vi "exampleloop_dirty.vi"() -> ()   [LabVIEW 2011]
uses:
  Kelvinox drivers/ITCAPPS - Copie.LLB/ITCSignal.ctl
  Kelvinox drivers/ITCAPPS - Copie.LLB/ITCSignals.ctl
  stopButton.vi
panel:
  in  "Refresh Rate [ms]":i32=1000 min=0
  out "Current sweep":dbl
  out "ITC ref":T1={"ITC"=0, "Signal"=enum."Sensor 3"}
  in  "Cancel run":bool
  out "DAC number":u8
  out "DAC":refnum<visa-resource-name>
  out "K2400 2":refnum<visa-resource-name>
  out "Lockin1":refnum<visa-resource-name>
  out "K2400 1":refnum<visa-resource-name>
  out "Priority type array":string[](array[string])
  out "Total sweep sequence":dbl[][](array[numeric])
  in  "Device Cluster":T3={"K2400 1"="", "K2400_1"=FALSE, "K2400 2"="", "K2400_2"=FALSE, "Lockin1"="", "Lockin1 present"=FALSE, "Lockin2"="", "Lockin2 present"=FALSE, "TIC"="", "Tcontrol"="OFF", "DMM1"="", "DMM1"=FALSE, "DMM2"="", "DMM2"=FALSE, "DAC"="", "DAC present"=FALSE, "DAC number"=0, "Bfield query"=FALSE, "Wvlen query"=FALSE, "ITC signal"={"ITC"=0, "Signal"=enum."Sensor 1"}}
  in  "Tab Control":T4(tab)
  in  "Loop Cluster":T5
  in  "START":bool
  in  "genTotalSequence":bool
  in  "Conversion Factor Fix\n1 V = ??":dbl=1.0
  in  "Fix type":string(combo)
  in  "Sweep Bias":dbl[](array[numeric])
  in  "Fix Bias":dbl[](array[numeric])
  in  "Priority sweep":i32=2
  in  "Priority fix":i32=2
  in  "sweep start [V]":dbl=-1.0 min=-200.0 max=200.0
  in  "sweep stop [V]":dbl=-5.0 min=-250.0 max=250.0
  in  "Nb steps":i32=800
  in  "sweep stop 2 [V]":dbl min=-250.0 max=250.0
  in  "Nb steps 2":i32
  in  "Nb Sweep":i32=1
  in  "Nb steps fix2":i32
  in  "Fix stop 2":dbl min=-250.0 max=250.0
  in  "Nb steps fix":i32=800
  in  "Fix stop":dbl=-5.0 min=-250.0 max=250.0
  in  "Fix start":dbl=-1.0 min=-200.0 max=200.0
  in  "genSweepArray":bool
  in  "genFixArray":bool
  in  "Sweep Instrument":string(combo)
  in  "Conversion Factor Sweep\n1 V = ??":dbl=1.0
  in  "Fix Instrument":string(combo)
  in  "Sweep type":string(combo)
  in  "T [K]":dbl[](array[numeric])
  in  "Priority T":i32=2
  in  "T stop [K] 2":dbl=-1.0 min=-200.0 max=200.0
  in  "Nb T steps 2":i32=800
  in  "Nb T steps":i32=800
  in  "T stop [K]":dbl=-1.0 min=-200.0 max=200.0
  in  "T start [K]":dbl=-1.0 min=-200.0 max=200.0
  in  "genTarray":bool
  in  "B [T]":dbl[](array[numeric])
  in  "Priority B":i32=2
  in  "B start [T]":dbl=-1.0 min=-200.0 max=200.0
  in  "B stop [T]":dbl=-1.0 min=-200.0 max=200.0
  in  "Rate [T/min]":dbl=-1.0 min=-200.0 max=200.0
  in  "Nb B steps":i32=800
  in  "Nb B steps 2":i32=800
  in  "B stop [T] 2":dbl=-1.0 min=-200.0 max=200.0
  in  "GenBarray":bool
  in  "File Basename":string
  out "Bias factor":dbl
  in  "SD bias [V]":dbl=-1.0 min=-200.0 max=200.0
  in  "Gain Cluster":T6={"Vsd"="Gate", "I 2probe 2"="Gate", "Vxy"="Gate", "Vxx"="Gate", "I leak BG"="Gate", "I leak TG"="Gate", "I Gain 1"=1000000.0, "V Gain 1"=1.0, "conversion factor BG"=1.0, "Vin / Vout 1"=1.0, "V Gain 2"=1.0, "Vin / Vout 2"=1.0, "V Gain 3"=1.0, "Vin / Vout 3"=1.0, "I Gain 2"=1000000.0, "I Gain 3"=1000000.0, "V BG"="Gate", "V TG"="Gate", "conversion factor TG"=1.0, "Vin / Vout 4"=1.0, "Vin / Vout 5"=1.0, "Manual Gain 1"=1.0, "Manual Gain 2"=1.0, "Manual Gain 3"=1.0} {"conversion factor TG" items=["1 V/V"=1.0, "4 V/V"=4.0, "15 V/V"=15.0, "30 V/V"=30.0, "45 V/V"=45.0]; "I Gain 3" items=["1"=1.0, "10"=10.0, "100"=100.0, "1K"=1000.0, "10K"=10000.0, "100K"=100000.0, "1M"=1000000.0, "10M"=10000000.0, "100M"=100000000.0, "1G"=1000000000.0]; "I Gain 2" items=["1"=1.0, "10"=10.0, "100"=100.0, "1K"=1000.0, "10K"=10000.0, "100K"=100000.0, "1M"=1000000.0, "10M"=10000000.0, "100M"=100000000.0, "1G"=1000000000.0]; "V Gain 3" items=["1"=1.0, "10"=10.0, "100"=100.0, "1K"=1000.0, "10K"=10000.0]; "V Gain 2" items=["1"=1.0, "10"=10.0, "100"=100.0, "1K"=1000.0, "10K"=10000.0]; "conversion factor BG" items=["1 V/V"=1.0, "4 V/V"=4.0, "15 V/V"=15.0, "30 V/V"=30.0, "45 V/V"=45.0]; "V Gain 1" items=["1"=1.0, "10"=10.0, "100"=100.0, "1K"=1000.0, "10K"=10000.0]; "I Gain 1" items=["1"=1.0, "10"=10.0, "100"=100.0, "1K"=1000.0, "10K"=10000.0, "100K"=100000.0, "1M"=1000000.0, "10M"=10000000.0, "100M"=100000000.0, "1G"=1000000000.0]}
  in  "Nb steps Increase 2":dbl=10.0
  in  "Gate Increase 2 (V)":dbl=0.1
  in  "Nb steps Increase":dbl=10.0
  in  "Gate Increase (V)":dbl=-0.1
  in  "Sweep back to zero":bool
  out "x .or. y?":bool
  in  "Step Delay (ms)":dbl=1000.0
  out "Total Progress":dbl(slide) scale=0.0..1.0
  in  "Nb Loop":i32
  out "Nb Loop Indicator":i32=2
  out "Nb Sweep Indicator":i32=3
  out "conversion factor sweep":dbl(ring)=1.0 items=["1 V/V"=1.0, "4 V/V"=4.0, "15 V/V"=15.0, "30 V/V"=30.0, "45 V/V"=45.0]
  in  "stop":bool
  in  "V step [V]":dbl=0.001
  in  "Folder Name":path=path "D:/users/marc/20180122_LiIon_EL/Freezing02/OutputHighT002p2.dat"
  # "Magnetic Field"
  # "Wavelength"
  # "IV Sweep Setting"
  # "IV Fix Setting"
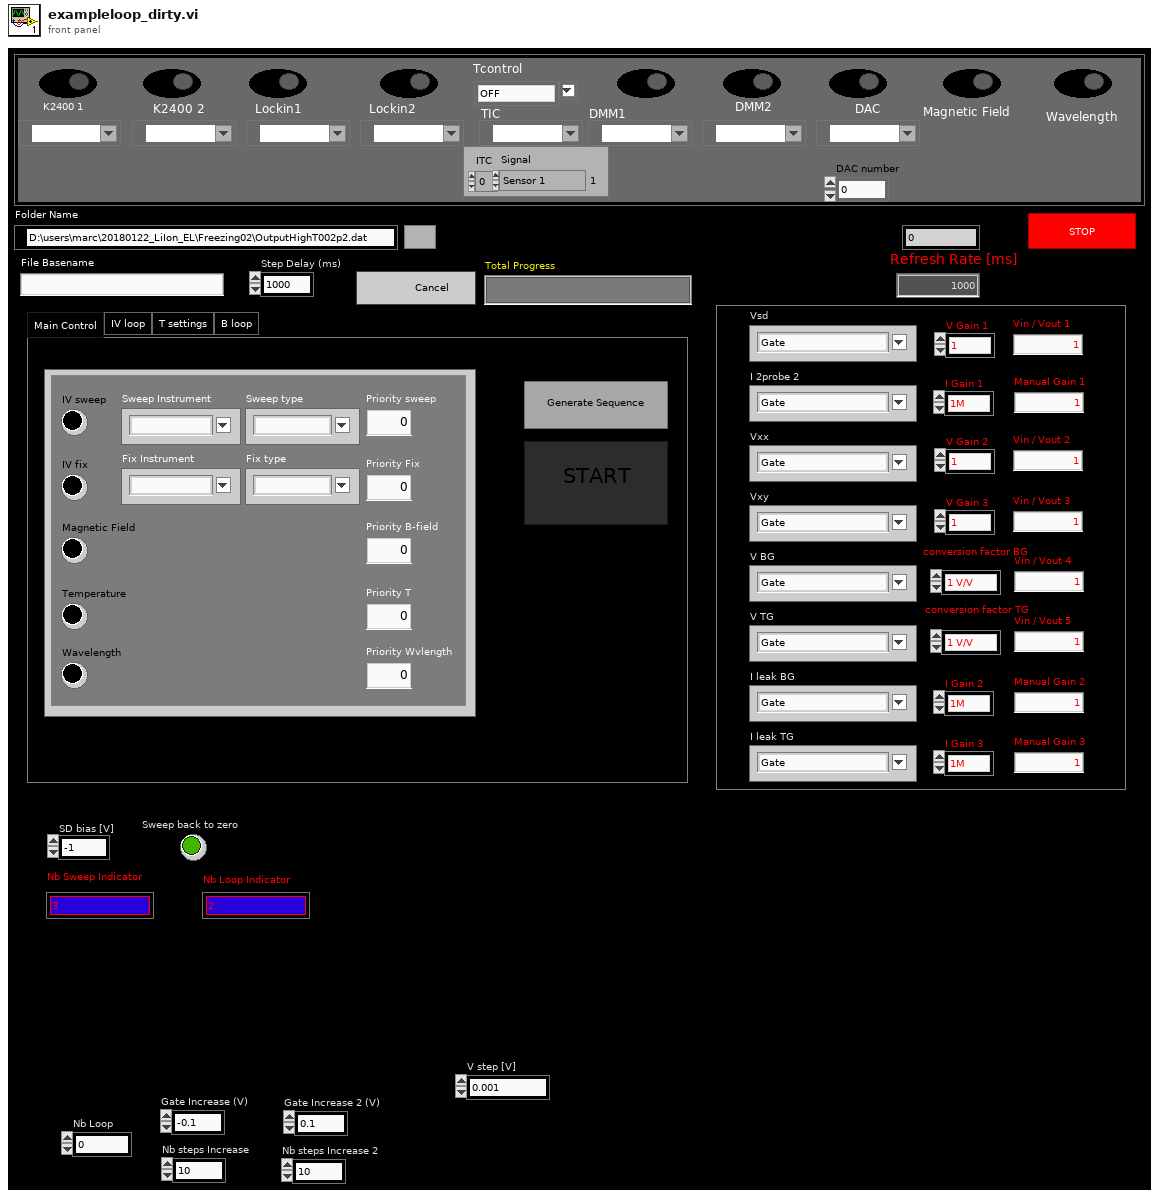
[diagram p1: front panel]
types:
  T1 = typedef "ITCSignal.ctl" = cluster{"ITC":u16, "Signal":T2}
  T2 = typedef "ITCSignals.ctl" = enum16{"Setpoint", "Sensor 1", "Sensor 2", "Sensor 3", "Needle Valve %", "Heater %"}
  T3 = cluster{"K2400 1":refnum<visa-resource-name>, "K2400_1":bool, "K2400 2":refnum<visa-resource-name>, "K2400_2":bool, "Lockin1":refnum<visa-resource-name>, "Lockin1 present":bool, "Lockin2":refnum<visa-resource-name>, "Lockin2 present":bool, "TIC":refnum<visa-resource-name>, "Tcontrol":string, "DMM1":refnum<visa-resource-name>, "DMM1":bool, "DMM2":refnum<visa-resource-name>, "DMM2":bool, "DAC":refnum<visa-resource-name>, "DAC present":bool, "DAC number":u8, "Bfield query":bool, "Wvlen query":bool, "ITC signal":T1}
  T4 = enum32{"Main Control", "IV loop", "T settings", "B loop"}
  T5 = cluster{"Sweep Instrument":string, "Sweep type":string, "Fix Instrument":string, "Fix type":string, "IV sweep":bool, "IV fix":bool, "Magnetic Field":bool, "Temperature":bool, "Wavelength":bool, "Priority sweep":dbl, "Priority Fix":dbl, "Priority B-field":dbl, "Priority T":dbl, "Priority Wvlength":dbl}
  T6 = cluster{"Vsd":string, "I 2probe 2":string, "Vxy":string, "Vxx":string, "I leak BG":string, "I leak TG":string, "I Gain 1":dbl, "V Gain 1":dbl, "conversion factor BG":dbl, "Vin / Vout 1":dbl, "V Gain 2":dbl, "Vin / Vout 2":dbl, "V Gain 3":dbl, "Vin / Vout 3":dbl, "I Gain 2":dbl, "I Gain 3":dbl, "V BG":string, "V TG":string, "conversion factor TG":dbl, "Vin / Vout 4":dbl, "Vin / Vout 5":dbl, "Manual Gain 1":dbl, "Manual Gain 2":dbl, "Manual Gain 3":dbl}
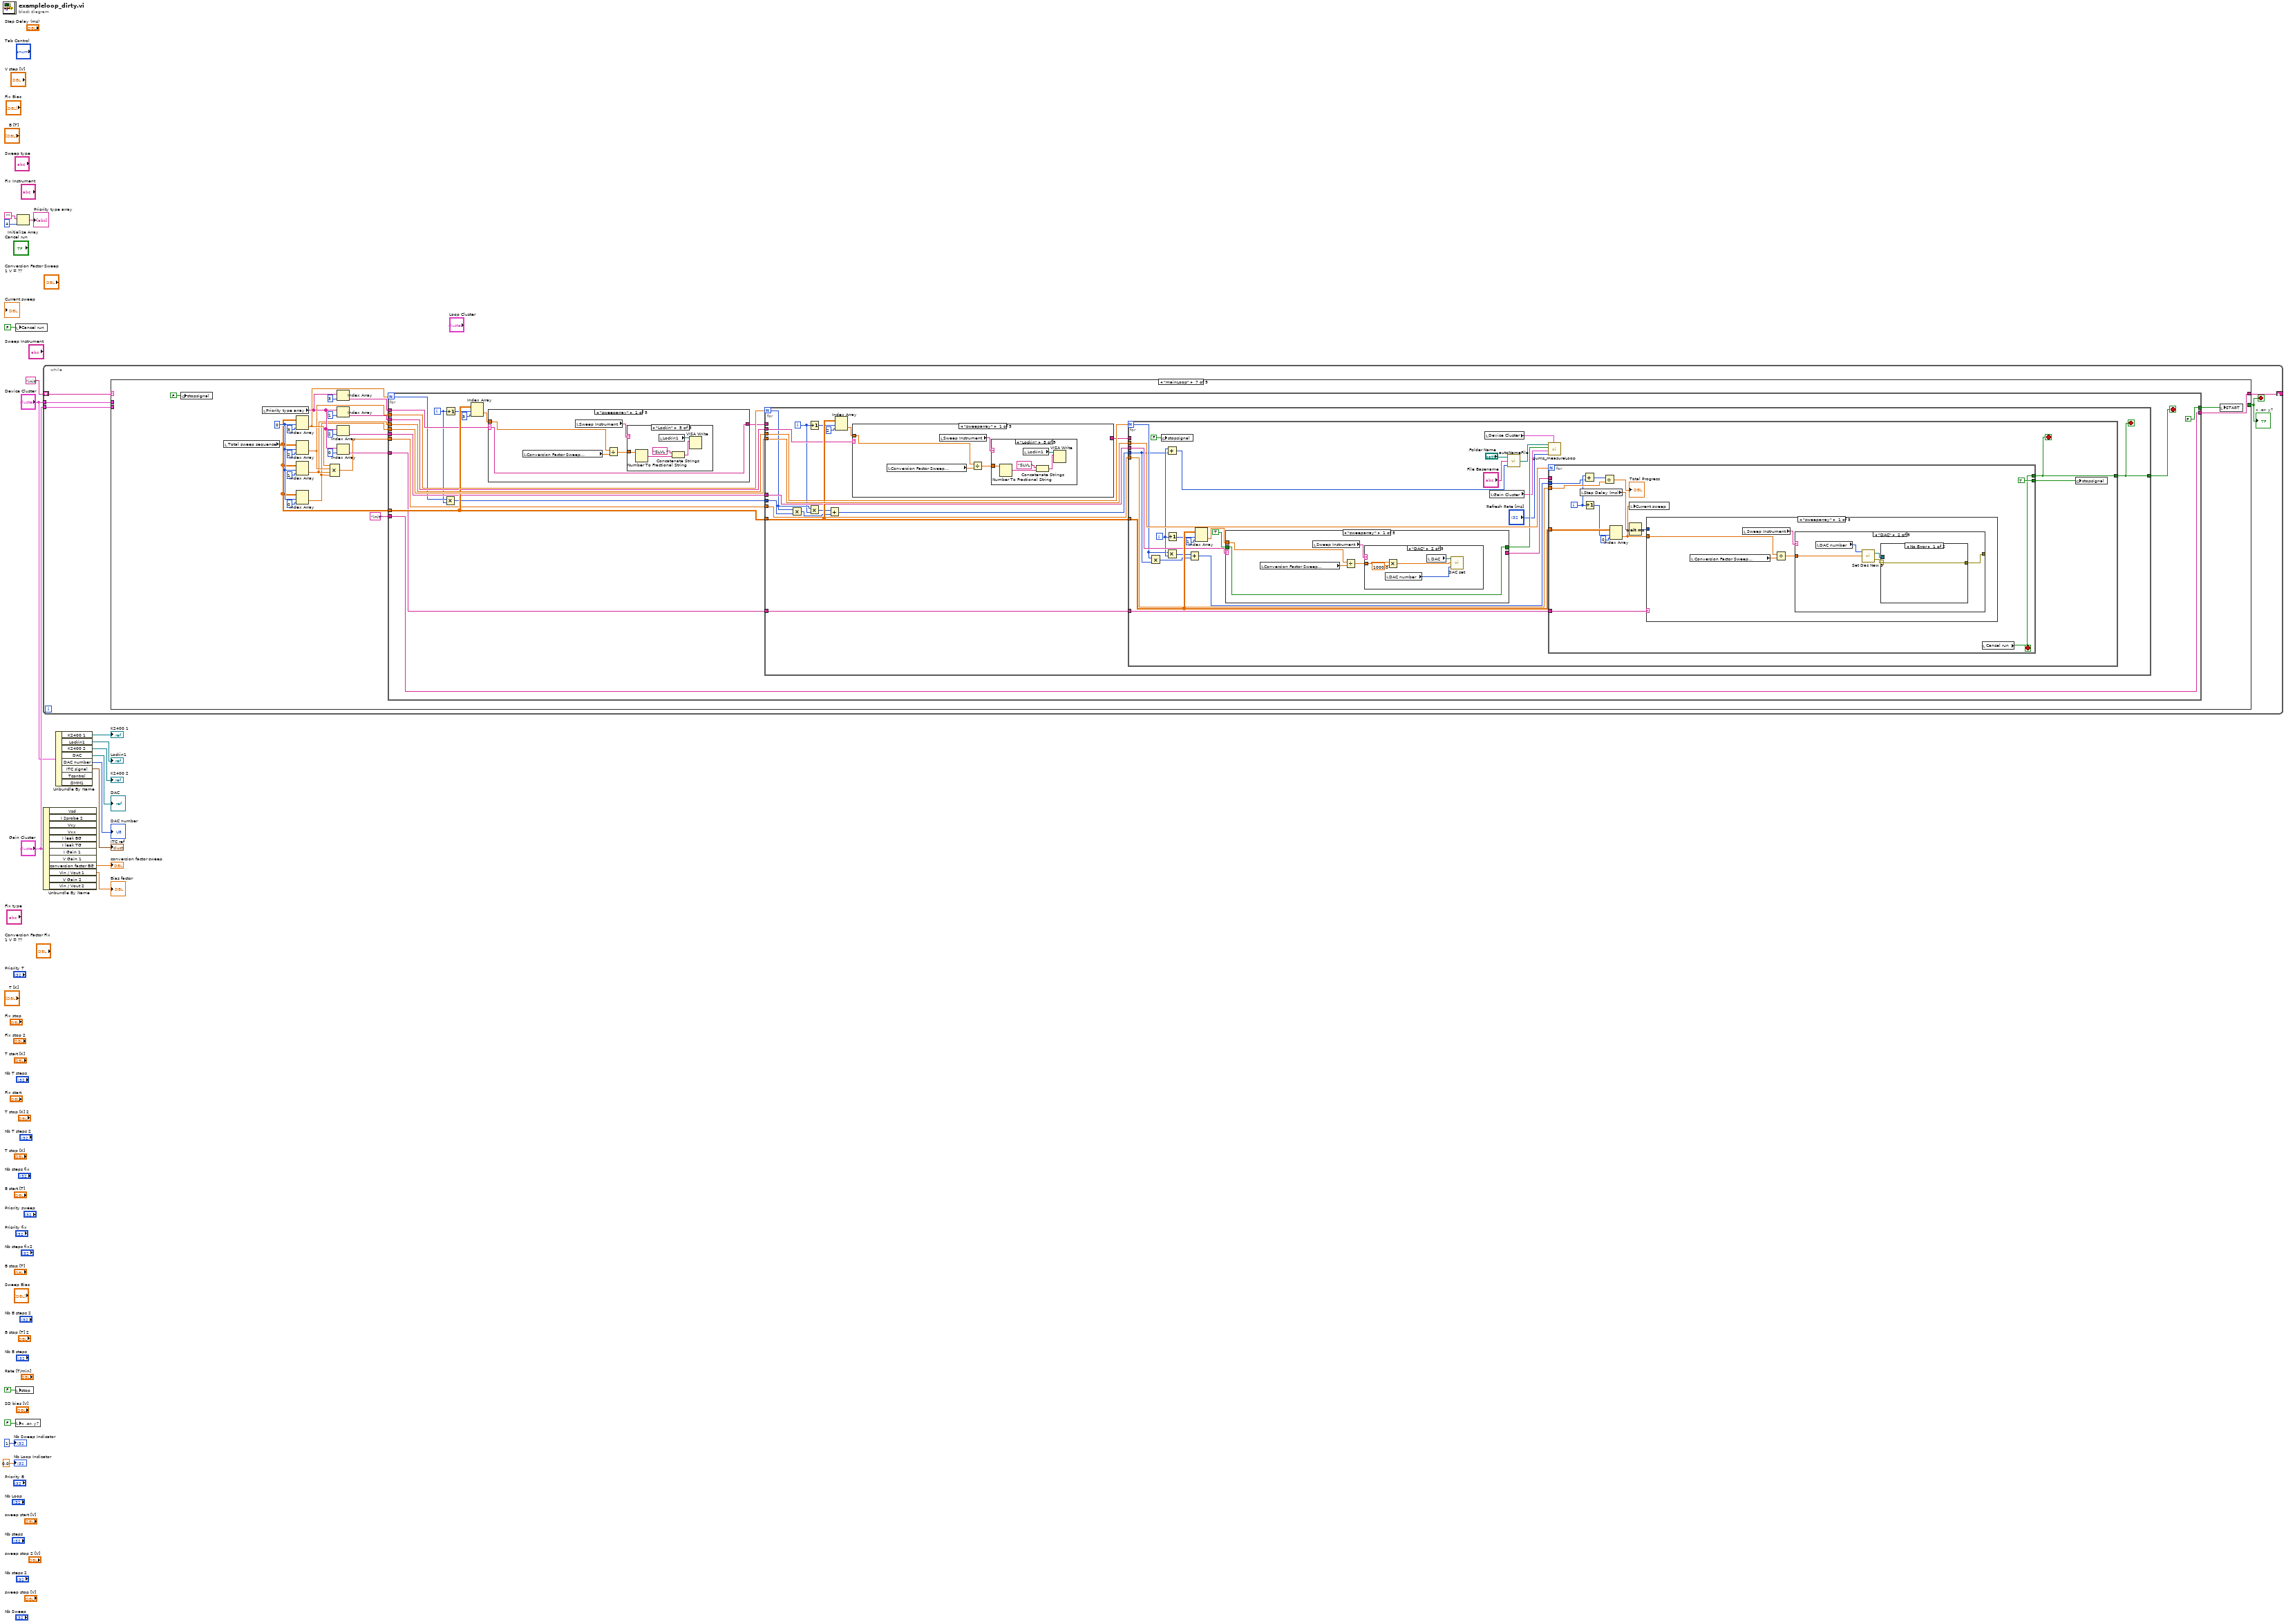
[diagram p0: block diagram]
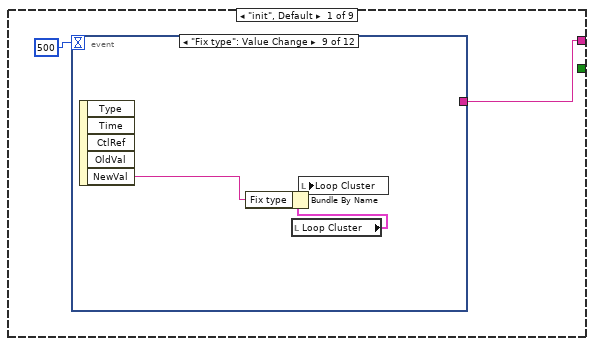
[diagram p2: hidden frame]
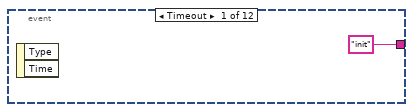
[diagram p3: hidden frame]
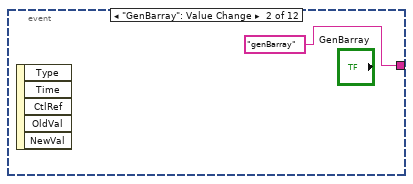
[diagram p4: hidden frame]
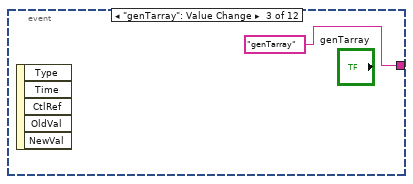
[diagram p5: hidden frame]
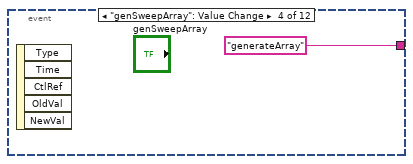
[diagram p6: hidden frame]
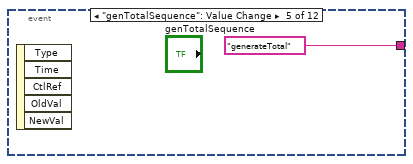
[diagram p7: hidden frame]
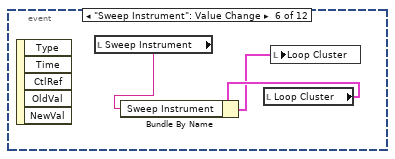
[diagram p8: hidden frame]
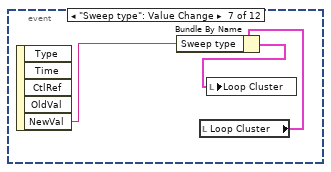
[diagram p9: hidden frame]
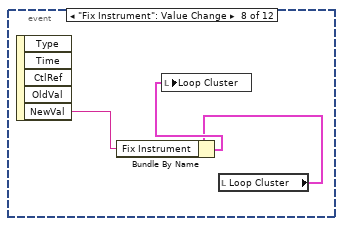
[diagram p10: hidden frame]
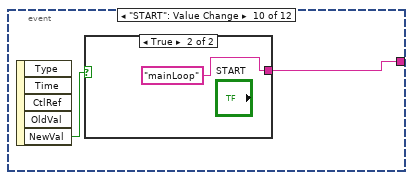
[diagram p11: hidden frame]
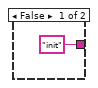
[diagram p12: hidden frame]
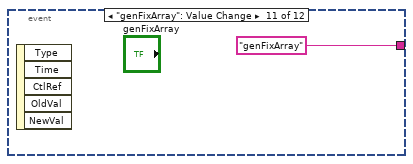
[diagram p13: hidden frame]
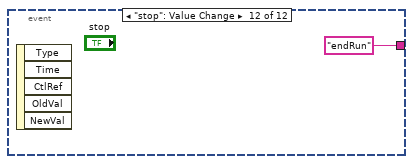
[diagram p14: hidden frame]
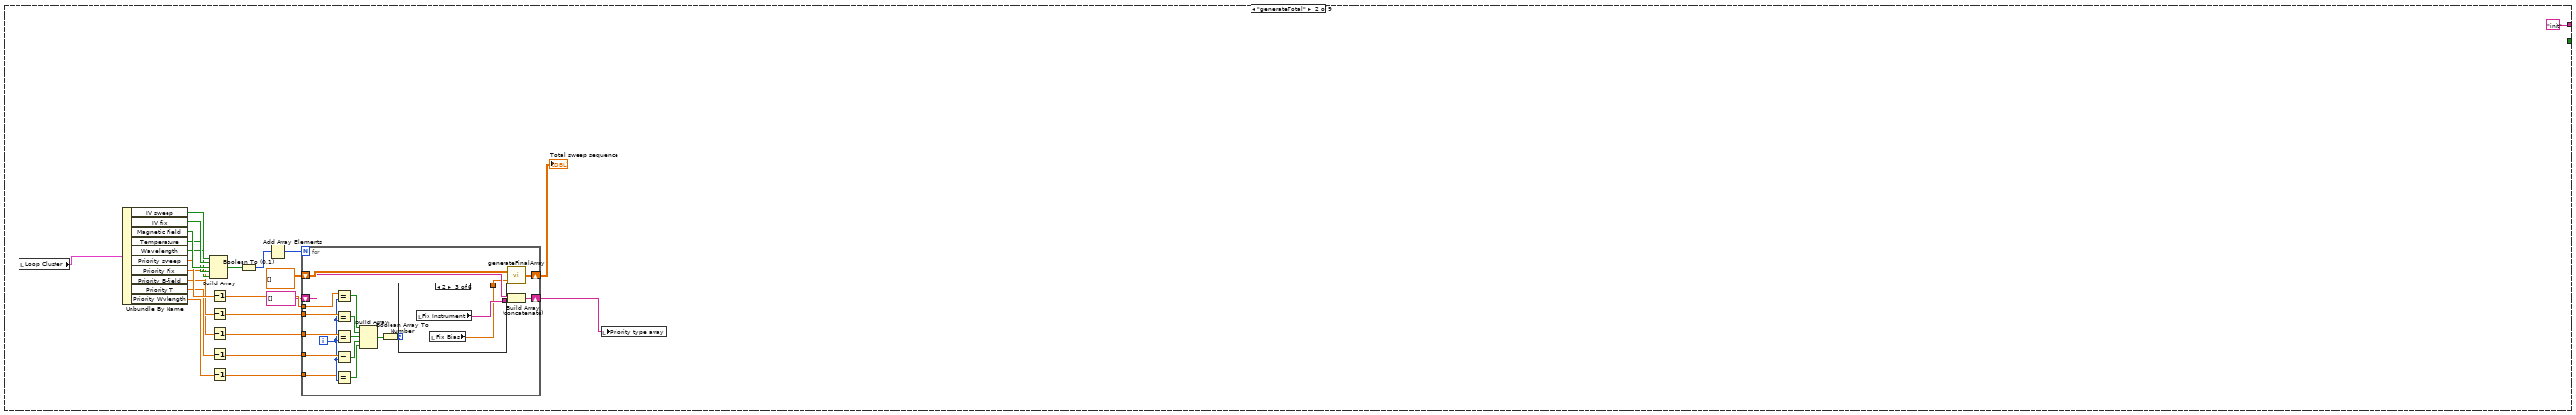
[diagram p15: hidden frame]
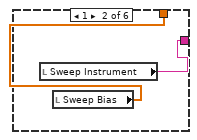
[diagram p17: hidden frame]
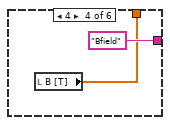
[diagram p18: hidden frame]
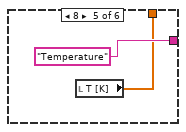
[diagram p19: hidden frame]
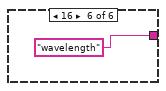
[diagram p20: hidden frame]
diagram:
  n1 = local write "Cancel run"(FALSE ("Cancel run")) -> ()
  n2 = local write "stop"(FALSE ("stop")) -> ()
  n3 = local write "x .or. y?"(FALSE ("x .or. y?")) -> ()
  n4 = Initialize Array("", 4 ("dimension size")) -> (→"Priority type array":string[])
  n5 = while {
    shift-right: [w20] -> _
    shift-left: "init" -> [w24]
    tunnel: "Gain Cluster" -> [w22]
    tunnel: "Device Cluster" -> [w21]
    stop <- w23 stop-if-true
    n6 = case shown="\"mainLoop\"" w24 {
      tunnel: [_ _ _ _ _ _ _ _ TRUE] -> w23
      tunnel: [w25 "init" "init" "init" "init" "init" w189 "generateArray" ""] -> w20
      tunnel: w22 -> [_ _ _ _ _ _ _ _ _]
      tunnel: w21 -> [_ _ _ _ _ _ _ _ _]
      frame "init", Default {
        n7 = event shown="[8] \"Fix type\": Value Change" {
          selector: _ -> [_ _ _ _ _ _ _ _ _ _ _ _]
          dyn-events: _ -> [_ _ _ _ _ _ _ _ _ _ _ _]
          timeout: 500 -> [_ _ _ _ _ _ _ _ _ _ _ _]
          tunnel: ["init" "genBarray" "genTarray" "generateArray" "generateTotal" _ _ _ _ w44 "genFixArray" "endRun"] -> w25
          event Timeout {
            n8 = event-data() -> ()  [unwired: 1 in, 2 out]
          }
          event "GenBarray": Value Change {
            n9 = event-data() -> ()  [unwired: 1 in, 5 out]
          }
          event "genTarray": Value Change {
            n10 = event-data() -> ()  [unwired: 1 in, 5 out]
          }
          event "genSweepArray": Value Change {
            n11 = event-data() -> ()  [unwired: 1 in, 5 out]
          }
          event "genTotalSequence": Value Change {
            n12 = event-data() -> ()  [unwired: 1 in, 5 out]
          }
          event "Sweep Instrument": Value Change {
            n13 = event-data() -> ()  [unwired: 1 in, 5 out]
            n14 = local read "Sweep Instrument"() -> (w33:string)
            n15 = local read "Loop Cluster"() -> (w34:T5)
            n16 = Bundle By Name(cluster=w34, "Sweep Instrument"=w33) -> (w32:T5)
            n17 = local write "Loop Cluster"(w32) -> ()
          }
          event "Sweep type": Value Change {
            n18 = event-data() -> ("NewVal"=w35:string)  [unwired: 1 in, 4 out]
            n19 = local read "Loop Cluster"() -> (w37:T5)
            n20 = Bundle By Name(cluster=w37, "Sweep type"=w35) -> (w36:T5)
            n21 = local write "Loop Cluster"(w36) -> ()
          }
          event "Fix Instrument": Value Change {
            n22 = event-data() -> ("NewVal"=w38:string)  [unwired: 1 in, 4 out]
            n23 = local read "Loop Cluster"() -> (w39:T5)
            n24 = Bundle By Name(cluster=w39, "Fix Instrument"=w38) -> (w40:T5)
            n25 = local write "Loop Cluster"(w40) -> ()
          }
          event "Fix type": Value Change {
            n26 = event-data() -> ("NewVal"=w43:string)  [unwired: 1 in, 4 out]
            n27 = local read "Loop Cluster"() -> (w42:T5)
            n28 = Bundle By Name(cluster=w42, "Fix type"=w43) -> (w41:T5)
            n29 = local write "Loop Cluster"(w41) -> ()
          }
          event "START": Value Change {
            n30 = event-data() -> ("NewVal"=w45:bool)  [unwired: 1 in, 4 out]
            n31 = case shown="True" w45 {
              tunnel: ["init" "mainLoop"] -> w44
              frame False {
              }
              frame True {
              }
            }
          }
          event "genFixArray": Value Change {
            n32 = event-data() -> ()  [unwired: 1 in, 5 out]
          }
          event "stop": Value Change {
            n33 = event-data() -> ()  [unwired: 1 in, 5 out]
          }
        }
      }
      frame "generateTotal" {
        n34 = local read "Loop Cluster"() -> (w52:T5)
        n35 = Unbundle By Name(w52) -> ("IV sweep"=w72:bool, "IV fix"=w71:bool, "Magnetic Field"=w70:bool, "Temperature"=w69:bool, "Wavelength"=w68:bool, "Priority sweep"=w63:dbl, "Priority Fix"=w62:dbl, "Priority B-field"=w61:dbl, "Priority T"=w60:dbl, "Priority Wvlength"=w55:dbl)
        n36 = Build Array(w72, w71, w70, w69, w68) -> (w66:bool[])
        n37 = Decrement(x=w63) -> (x-1=w56:dbl)
        n38 = Decrement(x=w62) -> (x-1=w57:dbl)
        n39 = Decrement(x=w61) -> (x-1=w58:dbl)
        n40 = Decrement(x=w60) -> (x-1=w59:dbl)
        n41 = Decrement(x=w55) -> (x-1=w54:dbl)
        n42 = Boolean To (0,1)(Boolean=w66) -> (0, 1=w67:i16[])
        n43 = Add Array Elements(numeric array=w67) -> (sum=w65:i16)
        n44 = for {
          N: w65 -> [_]
          shift-right: [w91] -> w51
          shift-left: dbl[][] [] ("Array In") -> [w92]
          tunnel: w59 -> [w88]
          tunnel: w58 -> [w89]
          tunnel: w57 -> [w90]
          tunnel: w56 -> [w82]
          tunnel: w54 -> [w84]
          shift-right: [w77] -> w50
          shift-left: string[] [] -> [w75]
          i -> [w85]
          n45 = Equal?(x=w82, y=w85) -> (x = y?=w81:bool)
          n46 = Equal?(x=w90, y=w85) -> (x = y?=w80:bool)
          n47 = Equal?(x=w89, y=w85) -> (x = y?=w79:bool)
          n48 = Equal?(x=w88, y=w85) -> (x = y?=w78:bool)
          n49 = Equal?(x=w84, y=w85) -> (x = y?=w83:bool)
          n50 = Build Array(w81, w80, w79, w78, w83) -> (w87:bool[])
          n51 = Boolean Array To Number(Boolean array=w87) -> (number=w86:u32)
          n52 = case shown="2" w86 {
            tunnel: [_ w94 w96 "Bfield" ("Fix Instrument") "Temperature" "wavelength"] -> w76
            tunnel: [_ w93 w95 w97 w99 _] -> w74
            frame 0, Default {
            }
            frame 1 {
              n53 = local read "Sweep Instrument"() -> (w94:string)
              n54 = local read "Sweep Bias"() -> (w93:dbl[])
            }
            frame 2 {
              n55 = local read "Fix Instrument"() -> (w96:string)
              n56 = local read "Fix Bias"() -> (w95:dbl[])
            }
            frame 4 {
              n57 = local read "B [T]"() -> (w97:dbl[])
            }
            frame 8 {
              n58 = local read "T [K]"() -> (w99:dbl[])
            }
            frame 16 {
            }
          }
          n59 = call "generateFinalArray.vi"("new array"=w74, "Array In"=w92) -> ("Array out"=w91:dbl[][])
          n60 = Build Array (concatenate)(w75, w76) -> (w77:string[])
        }
        "Total sweep sequence" <- w51
        n61 = local write "Priority type array"(w50) -> ()
      }
      frame "generateArray" {
        n62 = local read "Sweep Bias"() -> (w108:dbl[])
        n63 = local read "Nb Sweep"() -> (w109:i32)
        n64 = local read "Priority sweep"() -> (w102:i32)
        n65 = for {
          N: w109 -> [_]
          shift-right: [w113] -> w107
          shift-left: w108 -> [w112]
          n66 = local read "sweep stop 2 [V]"() -> (w115:dbl)
          n67 = local read "sweep start [V]"() -> (w116:dbl)
          n68 = local read "sweep stop [V]"() -> (w114:dbl)
          n69 = local read "Nb steps 2"() -> (w117:i32)
          n70 = local read "Nb steps"() -> (w118:i32)
          n71 = call "createLoopArray.vi"("Bgstop"=w114, "Bgstop2"=w115, "nbpoint1"=w118, "nbpoint2"=w117, "Bgstart"=w116) -> ("Outarray"=w111:dbl[])
          n72 = Build Array (concatenate)(w112, w111) -> (w113:dbl[])
        }
        n73 = local read "Priority type array"() -> (w106:string[])
        n74 = Decrement(x=w102) -> (x-1=w103:i32)
        n75 = Replace Array Subset(array=w106, new element="sweeparray" ("new element/subarray"), index=w103) -> (w105:string[])
        n76 = local write "Priority type array"(w105) -> ()
        n77 = local write "Sweep Bias"(w107) -> ()
      }
      frame "genFixArray" {
        n78 = local read "Priority fix"() -> (w119:i32)
        n79 = local read "Nb Sweep"() -> (w126:i32)
        n80 = local read "Fix Bias"() -> (w125:dbl[])
        n81 = local read "Priority type array"() -> (w123:string[])
        n82 = for {
          N: w126 -> [_]
          shift-right: [w130] -> w124
          shift-left: w125 -> [w129]
          n83 = local read "Nb steps fix2"() -> (w134:i32)
          n84 = local read "Nb steps fix"() -> (w135:i32)
          n85 = local read "Fix stop 2"() -> (w132:dbl)
          n86 = local read "Fix start"() -> (w133:dbl)
          n87 = local read "Fix stop"() -> (w131:dbl)
          n88 = call "createLoopArray.vi"("Bgstop"=w131, "Bgstop2"=w132, "nbpoint1"=w135, "nbpoint2"=w134, "Bgstart"=w133) -> ("Outarray"=w128:dbl[])
          n89 = Build Array (concatenate)(w129, w128) -> (w130:dbl[])
        }
        n90 = Decrement(x=w119) -> (x-1=w120:i32)
        n91 = Replace Array Subset(array=w123, new element="Fixarray" ("new element/subarray"), index=w120) -> (w122:string[])
        n92 = local write "Priority type array"(w122) -> ()
        n93 = local write "Fix Bias"(w124) -> ()
      }
      frame "genBarray" {
        n94 = local read "Priority B"() -> (w137:i32)
        n95 = local read "Priority type array"() -> (w140:string[])
        n96 = local read "Nb B steps 2"() -> (w143:i32)
        n97 = local read "B stop [T] 2"() -> (w145:dbl)
        n98 = local read "Nb B steps"() -> (w144:i32)
        n99 = local read "B start [T]"() -> (w147:dbl)
        n100 = local read "B stop [T]"() -> (w146:dbl)
        n101 = Decrement(x=w137) -> (x-1=w136:i32)
        n102 = Equal?(x=w137, y=1) -> (x = y?=w141:bool)
        n103 = case shown="True" w141 {
          tunnel: [w155 w156] -> w148
          tunnel: w147 -> [w154 w158]
          tunnel: w146 -> [w153 w157]
          tunnel: w145 -> [w152 _]
          tunnel: w144 -> [w151 _]
          tunnel: w143 -> [w150 _]
          frame False {
            n104 = call "createLoopArray.vi"("Bgstop"=w153, "Bgstop2"=w152, "nbpoint1"=w151, "nbpoint2"=w150, "Bgstart"=w154) -> ("Outarray"=w155:dbl[])
          }
          frame True {
            n105 = Build Array(w158, w157) -> (w156:dbl[])
          }
        }
        n106 = Replace Array Subset(array=w140, new element="Bfield" ("new element/subarray"), index=w136) -> (w139:string[])
        n107 = local write "Priority type array"(w139) -> ()
        n108 = local write "B [T]"(w148) -> ()
      }
      frame "genTarray" {
        n109 = local read "Priority T"() -> (w161:i32)
        n110 = local read "Priority type array"() -> (w163:string[])
        n111 = local read "Nb B steps 2"() -> (w166:i32)
        n112 = local read "B stop [T] 2"() -> (w168:dbl)
        n113 = local read "Nb B steps"() -> (w167:i32)
        n114 = local read "T start [K]"() -> (w170:dbl)
        n115 = local read "B stop [T]"() -> (w169:dbl)
        n116 = Decrement(x=w161) -> (x-1=w160:i32)
        n117 = Equal?(x=w161, y=1) -> (x = y?=w164:bool)
        n118 = case shown="True" w164 {
          tunnel: [w178 w179] -> w171
          tunnel: w170 -> [w177 w181]
          tunnel: w169 -> [w176 w180]
          tunnel: w168 -> [w175 _]
          tunnel: w167 -> [w174 _]
          tunnel: w166 -> [w173 _]
          frame False {
            n119 = call "createLoopArray.vi"("Bgstop"=w176, "Bgstop2"=w175, "nbpoint1"=w174, "nbpoint2"=w173, "Bgstart"=w177) -> ("Outarray"=w178:dbl[])
          }
          frame True {
            n120 = Build Array(w181, w180) -> (w179:dbl[])
          }
        }
        n121 = Replace Array Subset(array=w163, new element="Temperature" ("new element/subarray"), index=w160) -> (w162:string[])
        n122 = local write "Priority type array"(w162) -> ()
        n123 = local write "T [K]"(w171) -> ()
      }
      frame "mainLoop" {
        w203 = 0 ("index (row)")
        n124 = global write "stopButton.vi" "stopsignal"(FALSE ("stopsignal")) -> ()
        n125 = local read "Total sweep sequence"() -> (w199:dbl[][])
        n126 = local read "Priority type array"() -> (w198:string[])
        n127 = Index Array(array=w199, index (row)=w203, index (col)=3 ("index (row)")) -> (element=w187:dbl)
        n128 = Index Array(array=w199, index (row)=w203, index (col)=2 ("index (row)")) -> (element=w186:dbl)
        n129 = Index Array(array=w199, index (row)=w203, index (col)=1 ("index (row)")) -> (element=w185:dbl)
        n130 = Index Array(array=w199, index (row)=w203, index (col)=0 ("index (row)")) -> (element=w184:dbl)
        n131 = Compound Arithmetic op=MULTIPLY(w187, w186, w185, w184) -> (w183:dbl)
        n132 = Index Array(array=w198, index=3 ("index (row)")) -> (element=w193:string)
        n133 = Index Array(array=w198, index=1 ("index (row)")) -> (element=w192:string)
        n134 = Index Array(array=w198, index=2 ("index (row)")) -> (element=w191:string)
        n135 = Index Array(array=w198, index=0 ("index (row)")) -> (element=w190:string)
        n136 = for {
          N: w187 -> [w211]
          tunnel: w186 -> [w224]
          tunnel: w185 -> [w223]
          tunnel: w184 -> [w222]
          tunnel: w199 -> [w220]
          tunnel: w193 -> [w218]
          tunnel: w192 -> [w217]
          tunnel: w191 -> [w216]
          tunnel: w190 -> [w215]
          tunnel: [w213] -> w189
          tunnel: "init" -> [w213]
          tunnel: w183 -> [w208]
          tunnel: [FALSE] -> w182
          i -> [w210]
          stop <- w207 stop-if-true
          n137 = Multiply(x=w211, y=w210) -> (x*y=w209:i32)
          n138 = Increment(x=w210) -> (x+1=w212:i32)
          n139 = Index Array(array=w220, index (row)=w212, index (col)=3 ("disabled index (col)")) -> (element=w219:dbl)
          n140 = case shown="\"sweeparray\"" w218 {
            selector: w218 -> [w225 _ _ _ _]
            tunnel: w219 -> [w228 w242 _ w259 _]
            tunnel: [w225 _ _ _ _] -> w214
            frame "sweeparray" {
              n141 = local read "Conversion Factor Sweep\n1 V = ??"() -> (w229:dbl)
              n142 = local read "Sweep Instrument"() -> (w226:string)
              n143 = Divide(x=w228, y=w229) -> (x/y=w227:dbl)
              n144 = case shown="\"Lockin\"" w226 {
                tunnel: w227 -> [_ w230 w233 w234 w236]
                frame Default {
                }
                frame "DAC" {
                  n145 = Multiply(x=w230, y=1000.0) -> (x*y=w232:dbl)
                  n146 = call "DAC set.vi"("DAC set [mV]"=w232) -> ()  [unwired: 2 in, 1 out]
                }
                frame "K2400_2" {
                  n147 = call "K2400_ApplyVOLT_safe.vi"("Voltage target [V]"=w233) -> ()  [unwired: 2 in]
                }
                frame "K2400_1" {
                  n148 = call "K2400_ApplyVOLT_safe.vi"("Voltage target [V]"=w234) -> ()  [unwired: 2 in]
                }
                frame "Lockin" {
                  n149 = Number To Fractional String(number=w236) -> (F-format string=w239:string)  [unwired: 3 out]
                  n150 = local read "Lockin1"() -> (w235:refnum<visa-resource-name>)
                  n151 = Concatenate Strings("SLVL " ("chaîne"), w239) -> (w237:string)
                  n152 = VISA Write(VISA resource name=w235, write buffer=w237) -> ()  [unwired: 1 in, 3 out]
                }
              }
            }
            frame "Fixarray" {
              n153 = local read "Conversion Factor Fix\n1 V = ??"() -> (w243:dbl)
              n154 = local read "Fix Instrument"() -> (w240:string)
              n155 = Divide(x=w242, y=w243) -> (x/y=w241:dbl)
              n156 = case shown="\"K2400_1\"" w240 {
                tunnel: w241 -> [_ w246 w250 w252 w254]
                frame Default {
                }
                frame "DAC" {
                  n157 = local read "DAC number"() -> (w244:u8)
                  n158 = Multiply(x=w246, y=1000.0) -> (x*y=w248:dbl)
                  n159 = local read "DAC"() -> (w245:refnum<visa-resource-name>)
                  n160 = call "DAC set.vi"("DAC number"=w244, "DAC set [mV]"=w248, "DAC COM port"=w245) -> ()  [unwired: 1 out]
                }
                frame "K2400_2" {
                  n161 = local read "K2400 2"() -> (w249:refnum<visa-resource-name>)
                  n162 = call "K2400_ApplyVOLT_safe.vi"("Voltage target [V]"=w250, "VISA Resource Name"=w249) -> ()  [unwired: 1 in]
                }
                frame "K2400_1" {
                  n163 = local read "K2400 1"() -> (w251:refnum<visa-resource-name>)
                  n164 = call "K2400_ApplyVOLT_safe.vi"("Voltage target [V]"=w252, "VISA Resource Name"=w251) -> ()  [unwired: 1 in]
                }
                frame "Lockin" {
                  n165 = Number To Fractional String(number=w254) -> (F-format string=w257:string)  [unwired: 3 out]
                  n166 = local read "Lockin1"() -> (w253:refnum<visa-resource-name>)
                  n167 = Concatenate Strings("SLVL " ("chaîne"), w257) -> (w255:string)
                  n168 = VISA Write(VISA resource name=w253, write buffer=w255) -> ()  [unwired: 1 in, 3 out]
                }
              }
            }
            frame Default {
            }
            frame "Bfield" {
              n169 = node(w259) -> (w258:dbl[unit])
              n170 = local read "Rate [T/min]"() -> (w260:dbl)
              n171 = node(w260) -> (w261:dbl[unit])
              n172 = call "TeslSetField.vi"("Sweep rate"=w261, "Field required:"=w258) -> ()  [unwired: 2 in, 2 out]
            }
            frame "Temperature" {
              n173 = local read "ITC ref"() -> (w262:T1)
              n174 = call "Tloop.vi"("ITCSignal"=w262, "Regulate ?"=TRUE) -> ()  [unwired: 3 in, 2 out]
            }
          }
          n175 = for {
            N: w224 -> [w270]
            tunnel: w223 -> [w281]
            tunnel: w222 -> [w280]
            tunnel: w220 -> [w279]
            tunnel: w217 -> [w276]
            tunnel: w216 -> [w275]
            tunnel: w215 -> [w274]
            tunnel: w214 -> [_]
            tunnel: w209 -> [w271]
            tunnel: w208 -> [w265]
            tunnel: [w264] -> w207
            i -> [w269]
            stop <- w264 stop-if-true
            n176 = Multiply(x=w270, y=w271) -> (x*y=w267:i32)
            n177 = Increment(x=w269) -> (x+1=w272:i32)
            n178 = Multiply(x=w270, y=w269) -> (x*y=w268:i32)
            n179 = Add(x=w268, y=w267) -> (x+y=w266:i32)
            n180 = Index Array(array=w279, index (row)=w272, index (col)=2 ("disabled index (col)")) -> (element=w277:dbl)
            n181 = case shown="\"sweeparray\"" w276 {
              selector: w276 -> [_ w296 _ _ _]
              tunnel: w277 -> [w284 w299 _ w316 _]
              tunnel: [_ w296 _ _ _] -> w273
              frame "sweeparray" {
                n182 = local read "Conversion Factor Sweep\n1 V = ??"() -> (w285:dbl)
                n183 = local read "Sweep Instrument"() -> (w282:string)
                n184 = Divide(x=w284, y=w285) -> (x/y=w283:dbl)
                n185 = case shown="\"Lockin\"" w282 {
                  tunnel: w283 -> [_ w286 w289 w290 w292]
                  frame Default {
                  }
                  frame "DAC" {
                    n186 = Multiply(x=w286, y=1000.0) -> (x*y=w288:dbl)
                    n187 = call "DAC set.vi"("DAC set [mV]"=w288) -> ()  [unwired: 2 in, 1 out]
                  }
                  frame "K2400_2" {
                    n188 = call "K2400_ApplyVOLT_safe.vi"("Voltage target [V]"=w289) -> ()  [unwired: 2 in]
                  }
                  frame "K2400_1" {
                    n189 = call "K2400_ApplyVOLT_safe.vi"("Voltage target [V]"=w290) -> ()  [unwired: 2 in]
                  }
                  frame "Lockin" {
                    n190 = Number To Fractional String(number=w292) -> (F-format string=w295:string)  [unwired: 3 out]
                    n191 = local read "Lockin1"() -> (w291:refnum<visa-resource-name>)
                    n192 = Concatenate Strings("SLVL " ("chaîne"), w295) -> (w293:string)
                    n193 = VISA Write(VISA resource name=w291, write buffer=w293) -> ()  [unwired: 1 in, 3 out]
                  }
                }
              }
              frame "Fixarray" {
                n194 = local read "Conversion Factor Fix\n1 V = ??"() -> (w300:dbl)
                n195 = local read "Fix Instrument"() -> (w297:string)
                n196 = Divide(x=w299, y=w300) -> (x/y=w298:dbl)
                n197 = case shown="\"Lockin\"" w297 {
                  tunnel: w298 -> [_ w303 w307 w309 w311]
                  frame Default {
                  }
                  frame "DAC" {
                    n198 = local read "DAC number"() -> (w302:u8)
                    n199 = Multiply(x=w303, y=1000.0) -> (x*y=w305:dbl)
                    n200 = local read "DAC"() -> (w301:refnum<visa-resource-name>)
                    n201 = call "DAC set.vi"("DAC number"=w302, "DAC set [mV]"=w305, "DAC COM port"=w301) -> ()  [unwired: 1 out]
                  }
                  frame "K2400_2" {
                    n202 = local read "K2400 2"() -> (w306:refnum<visa-resource-name>)
                    n203 = call "K2400_ApplyVOLT_safe.vi"("Voltage target [V]"=w307, "VISA Resource Name"=w306) -> ()  [unwired: 1 in]
                  }
                  frame "K2400_1" {
                    n204 = local read "K2400 1"() -> (w308:refnum<visa-resource-name>)
                    n205 = call "K2400_ApplyVOLT_safe.vi"("Voltage target [V]"=w309, "VISA Resource Name"=w308) -> ()  [unwired: 1 in]
                  }
                  frame "Lockin" {
                    n206 = Number To Fractional String(number=w311) -> (F-format string=w314:string)  [unwired: 3 out]
                    n207 = local read "Lockin1"() -> (w310:refnum<visa-resource-name>)
                    n208 = Concatenate Strings("SLVL " ("chaîne"), w314) -> (w312:string)
                    n209 = VISA Write(VISA resource name=w310, write buffer=w312) -> ()  [unwired: 1 in, 3 out]
                  }
                }
              }
              frame Default {
              }
              frame "Bfield" {
                n210 = node(w316) -> (w315:dbl[unit])
                n211 = local read "Rate [T/min]"() -> (w317:dbl)
                n212 = node(w317) -> (w318:dbl[unit])
                n213 = call "TeslSetField.vi"("Sweep rate"=w318, "Field required:"=w315) -> ()  [unwired: 2 in, 2 out]
              }
              frame "Temperature" {
                n214 = local read "ITC ref"() -> (w319:T1)
                n215 = call "Tloop.vi"("ITCSignal"=w319, "Regulate ?"=TRUE) -> ()  [unwired: 3 in, 2 out]
              }
            }
            n216 = for {
              N: w281 -> [w327]
              tunnel: w280 -> [w344]
              tunnel: w279 -> [w341]
              tunnel: w275 -> [w339]
              tunnel: w274 -> [w338]
              tunnel: w273 -> [_]
              tunnel: w266 -> [w326]
              tunnel: w265 -> [w330]
              tunnel: [w322] -> w264
              i -> [w328]
              stop <- w322 stop-if-true
              n217 = Multiply(x=w327, y=w326) -> (x*y=w324:i32)
              n218 = global write "stopButton.vi" "stopsignal"(FALSE) -> ()
              n219 = Add(x=w328, y=w326) -> (x+y=w331:i32)
              n220 = Multiply(x=w327, y=w328) -> (x*y=w325:i32)
              n221 = Increment(x=w328) -> (x+1=w332:i32)
              n222 = Add(x=w325, y=w324) -> (x+y=w323:i32)
              n223 = Index Array(array=w341, index (row)=w332, index (col)=1 ("disabled index (col)")) -> (element=w340:dbl)
              n224 = case shown="\"sweeparray\"" w339 {
                selector: w339 -> [_ _ w382 _ _]
                tunnel: w340 -> [w351 w370 _ w386 _]
                tunnel: TRUE ("SaveDataQuery") -> [w348 w367 w383 w384 w391]
                tunnel: [w348 w367 w383 w384 w391] -> w336
                tunnel: [_ _ w382 _ _] -> w335
                frame "sweeparray" {
                  n225 = local read "Conversion Factor Sweep\n1 V = ??"() -> (w352:dbl)
                  n226 = local read "Sweep Instrument"() -> (w349:string)
                  n227 = Divide(x=w351, y=w352) -> (x/y=w350:dbl)
                  n228 = case shown="\"DAC\"" w349 {
                    tunnel: w350 -> [_ w355 w359 w361 w363]
                    frame Default {
                    }
                    frame "DAC" {
                      n229 = local read "DAC number"() -> (w353:u8)
                      n230 = Multiply(x=w355, y=1000.0) -> (x*y=w357:dbl)
                      n231 = local read "DAC"() -> (w354:refnum<visa-resource-name>)
                      n232 = call "DAC set.vi"("DAC number"=w353, "DAC set [mV]"=w357, "DAC COM port"=w354) -> ()  [unwired: 1 out]
                    }
                    frame "K2400_2" {
                      n233 = local read "K2400 2"() -> (w358:refnum<visa-resource-name>)
                      n234 = call "K2400_ApplyVOLT_safe.vi"("Voltage target [V]"=w359, "VISA Resource Name"=w358) -> ()  [unwired: 1 in]
                    }
                    frame "K2400_1" {
                      n235 = local read "K2400 1"() -> (w360:refnum<visa-resource-name>)
                      n236 = call "K2400_ApplyVOLT_safe.vi"("Voltage target [V]"=w361, "VISA Resource Name"=w360) -> ()  [unwired: 1 in]
                    }
                    frame "Lockin" {
                      n237 = Number To Fractional String(number=w363) -> (F-format string=w366:string)  [unwired: 3 out]
                      n238 = local read "Lockin1"() -> (w362:refnum<visa-resource-name>)
                      n239 = Concatenate Strings("SLVL " ("chaîne"), w366) -> (w364:string)
                      n240 = VISA Write(VISA resource name=w362, write buffer=w364) -> ()  [unwired: 1 in, 3 out]
                    }
                  }
                }
                frame "Fixarray" {
                  n241 = local read "Conversion Factor Fix\n1 V = ??"() -> (w371:dbl)
                  n242 = local read "Fix Instrument"() -> (w368:string)
                  n243 = Divide(x=w370, y=w371) -> (x/y=w369:dbl)
                  n244 = case shown="\"Lockin\"" w368 {
                    tunnel: w369 -> [_ w372 w375 w376 w378]
                    frame Default {
                    }
                    frame "DAC" {
                      n245 = Multiply(x=w372, y=1000.0) -> (x*y=w374:dbl)
                      n246 = call "DAC set.vi"("DAC set [mV]"=w374) -> ()  [unwired: 2 in, 1 out]
                    }
                    frame "K2400_2" {
                      n247 = call "K2400_ApplyVOLT_safe.vi"("Voltage target [V]"=w375) -> ()  [unwired: 2 in]
                    }
                    frame "K2400_1" {
                      n248 = call "K2400_ApplyVOLT_safe.vi"("Voltage target [V]"=w376) -> ()  [unwired: 2 in]
                    }
                    frame "Lockin" {
                      n249 = Number To Fractional String(number=w378) -> (F-format string=w381:string)  [unwired: 3 out]
                      n250 = local read "Lockin1"() -> (w377:refnum<visa-resource-name>)
                      n251 = Concatenate Strings("SLVL " ("chaîne"), w381) -> (w379:string)
                      n252 = VISA Write(VISA resource name=w377, write buffer=w379) -> ()  [unwired: 1 in, 3 out]
                    }
                  }
                }
                frame Default {
                }
                frame "Bfield" {
                  n253 = node(w386) -> (w385:dbl[unit])
                  n254 = local read "Rate [T/min]"() -> (w387:dbl)
                  n255 = node(w387) -> (w388:dbl[unit])
                  n256 = call "TeslSetField.vi"("Sweep rate"=w388, "Field required:"=w385) -> ()  [unwired: 2 in, 2 out]
                }
                frame "Temperature" {
                  n257 = local read "ITC ref"() -> (w389:T1)
                  n258 = call "Tloop.vi"("ITCSignal"=w389, "Regulate ?"=TRUE) -> ()  [unwired: 3 in, 2 out]
                }
              }
              n259 = local read "Device Cluster"() -> (w334:T3)
              n260 = local read "Gain Cluster"() -> (w333:T6)
              n261 = call "autoNameFile.vi"("num"=w331, "File Basename"="File Basename", "Folder Name"="Folder Name") -> ("path"=w347:path)
              n262 = call "gums_measureLoop.vi"("File Name"=w347, "SaveDataQuery"=w336, "Gain Cluster 2"=w333, "Refresh Rate [ms]"="Refresh Rate [ms]", "Device Cluster"=w334) -> ()  [unwired: 6 in]
              n263 = for {
                N: w344 -> [_]
                tunnel: [TRUE ("stopsignal")] -> w343
                tunnel: w341 -> [w404]
                tunnel: w338 -> [w402]
                tunnel: w335 -> [_]
                tunnel: w330 -> [w400]
                tunnel: w323 -> [w397]
                tunnel: [w395] -> w322
                i -> [w398]
                stop <- w395 stop-if-true
                n264 = local read "Step Delay (ms)"() -> (w393:dbl)
                n265 = Add(x=w398, y=w397) -> (x+y=w396:i32)
                n266 = Increment(x=w398) -> (x+1=w401:i32)
                n267 = Divide(x=w396, y=w400) -> (x/y=→"Total Progress":dbl)
                n268 = Index Array(array=w404, index (row)=w401, index (col)=0 ("disabled index (col)")) -> (element=w394:dbl)
                n269 = local write "Current sweep"(w394) -> ()
                n270 = Wait (ms)(milliseconds to wait=w393) -> (millisecond timer value=w392:u32)
                n271 = case shown="\"sweeparray\"" w402 {
                  tunnel: w394 -> [w408 w433 _ w450 w454]
                  tunnel: w392 -> [_ _ _ _ _]
                  frame "sweeparray" {
                    n272 = local read "Conversion Factor Sweep\n1 V = ??"() -> (w409:dbl)
                    n273 = local read "Sweep Instrument"() -> (w406:string)
                    n274 = Divide(x=w408, y=w409) -> (x/y=w407:dbl)
                    n275 = case shown="\"DAC\"" w406 {
                      tunnel: w407 -> [_ w413 w421 w424 w427]
                      tunnel: [_ w410 _ w422 w425] -> _
                      frame Default {
                      }
                      frame "DAC" {
                        n276 = local read "DAC number"() -> (w414:u8)
                        n277 = call "Set Dac New 3.vi"("DATA (V)"=w413, "DAC nr"=w414) -> ("error out"=w412:errorcluster, "VISA resource name OUT"=w411:refnum<visa-resource-name>)  [unwired: 1 in]
                        n278 = case shown="No Error" w412 {
                          selector: w412 -> [w415 _]
                          tunnel: w411 -> [_ w418]
                          tunnel: [w415 w416] -> w410
                          frame No Error {
                          }
                          frame Error {
                            n279 = flat-sequence {
                              tunnel: w418 -> [w419]
                              tunnel: [w419] -> w417
                              frame #0 {
                                n280 = call "closeRS232.vi"("VISA resource name"=w419) -> ()  [unwired: 2 in]
                              }
                            }
                            n281 = call "openRS232.vi"("com"=w417) -> ("error out"=w416:errorcluster)  [unwired: 1 out]
                          }
                        }
                      }
                      frame "K2400_2" {
                        n282 = local read "K2400 2"() -> (w420:refnum<visa-resource-name>)
                        n283 = call "K2400setV.vi"("Voltage target [V]"=w421, "VISA Resource Name"=w420) -> ()  [unwired: 1 in, 2 out]
                      }
                      frame "K2400_1" {
                        n284 = local read "K2400 1"() -> (w423:refnum<visa-resource-name>)
                        n285 = call "K2400setV.vi"("Voltage target [V]"=w424, "VISA Resource Name"=w423) -> ("error out"=w422:errorcluster)  [unwired: 1 in, 1 out]
                      }
                      frame "Lockin" {
                        n286 = Number To Fractional String(number=w427) -> (F-format string=w430:string)  [unwired: 3 out]
                        n287 = local read "Lockin1"() -> (w426:refnum<visa-resource-name>)
                        n288 = Concatenate Strings("SLVL " ("chaîne"), w430) -> (w428:string)
                        n289 = VISA Write(VISA resource name=w426, write buffer=w428) -> (error out=w425:errorcluster)  [unwired: 1 in, 2 out]
                      }
                    }
                  }
                  frame "Fixarray" {
                    n290 = local read "Conversion Factor Fix\n1 V = ??"() -> (w434:dbl)
                    n291 = local read "Fix Instrument"() -> (w431:string)
                    n292 = Divide(x=w433, y=w434) -> (x/y=w432:dbl)
                    n293 = case shown="\"Lockin\"" w431 {
                      tunnel: w432 -> [_ w437 w441 w443 w445]
                      frame Default {
                      }
                      frame "DAC" {
                        n294 = local read "DAC number"() -> (w435:u8)
                        n295 = Multiply(x=w437, y=1000.0) -> (x*y=w439:dbl)
                        n296 = local read "DAC"() -> (w436:refnum<visa-resource-name>)
                        n297 = call "DAC set.vi"("DAC number"=w435, "DAC set [mV]"=w439, "DAC COM port"=w436) -> ()  [unwired: 1 out]
                      }
                      frame "K2400_2" {
                        n298 = local read "K2400 2"() -> (w440:refnum<visa-resource-name>)
                        n299 = call "K2400_ApplyVOLT_safe.vi"("Voltage target [V]"=w441, "VISA Resource Name"=w440) -> ()  [unwired: 1 in]
                      }
                      frame "K2400_1" {
                        n300 = local read "K2400 1"() -> (w442:refnum<visa-resource-name>)
                        n301 = call "K2400_ApplyVOLT_safe.vi"("Voltage target [V]"=w443, "VISA Resource Name"=w442) -> ()  [unwired: 1 in]
                      }
                      frame "Lockin" {
                        n302 = Number To Fractional String(number=w445) -> (F-format string=w448:string)  [unwired: 3 out]
                        n303 = local read "Lockin1"() -> (w444:refnum<visa-resource-name>)
                        n304 = Concatenate Strings("SLVL " ("chaîne"), w448) -> (w446:string)
                        n305 = VISA Write(VISA resource name=w444, write buffer=w446) -> ()  [unwired: 1 in, 3 out]
                      }
                    }
                  }
                  frame Default {
                  }
                  frame "Bfield" {
                    n306 = node(w450) -> (w449:dbl[unit])
                    n307 = local read "Rate [T/min]"() -> (w451:dbl)
                    n308 = node(w451) -> (w452:dbl[unit])
                    n309 = call "TeslSetField.vi"("Sweep rate"=w452, "Field required:"=w449) -> ()  [unwired: 2 in, 2 out]
                  }
                  frame "Temperature" {
                    n310 = local read "ITC ref"() -> (w455:T1)
                    n311 = call "Tloop.vi"("ITCSignal"=w455, "T target [K]"=w454, "Regulate ?"=TRUE) -> ()  [unwired: 2 in, 2 out]
                  }
                }
                n312 = local read "Cancel run"() -> (w395:bool)
              }
              n313 = global write "stopButton.vi" "stopsignal"(w343) -> ()
            }
          }
        }
        n314 = local write "START"(w182) -> ()
      }
      frame "loopIncrease" {
        w468 = 1 ("Nb Sweep Indicator")
        n315 = local read "Nb Loop Indicator"() -> (w471:i32)
        n316 = local write "Priority B"(w468) -> ()
        n317 = local write "Nb Sweep Indicator"(w468) -> ()
        n318 = local read "sweep stop 2 [V]"() -> (w464:dbl)
        n319 = local read "sweep stop [V]"() -> (w466:dbl)
        n320 = local read "Nb steps 2"() -> (w463:i32)
        n321 = local read "Nb steps"() -> (w462:i32)
        n322 = Add(x="Nb steps Increase", y=w462) -> (x+y=w458:dbl)
        n323 = Add(x="Nb steps Increase 2", y=w463) -> (x+y=w459:dbl)
        n324 = Add(x=w464, y="Gate Increase 2 (V)") -> (x+y=w456:dbl)
        n325 = Add(x="Gate Increase (V)", y=w466) -> (x+y=w457:dbl)
        n326 = Increment(x=w471) -> (x+1=w470:i32)
        n327 = local write "Nb steps"(w458) -> ()
        n328 = local write "Nb Loop Indicator"(w470) -> ()
        n329 = local write "Nb steps 2"(w459) -> ()
        n330 = local write "sweep stop 2 [V]"(w456) -> ()
        n331 = local write "sweep stop [V]"(w457) -> ()
      }
      frame "endRun" {
        n332 = case shown="True" "Sweep back to zero" {
          frame False {
          }
          frame True {
            n333 = local read "V step [V]"() -> (w475:dbl)
            n334 = call "K2400_ApplyVOLT_safe.vi"("V step [V]"=w475, "Voltage target [V]"=0.0) -> ()  [unwired: 1 in]
          }
        }
      }
    }
    "x .or. y?" <- w23
  }
  n335 = Unbundle By Name("Gain Cluster") -> ("conversion factor BG"=→"conversion factor sweep":dbl, "Vin / Vout 1"=→"Bias factor":dbl)  [unwired: 10 out]
  n336 = Unbundle By Name("Device Cluster") -> ("K2400 1"=→"K2400 1":refnum<visa-resource-name>, "Lockin1"=→"Lockin1":refnum<visa-resource-name>, "K2400 2"=→"K2400 2":refnum<visa-resource-name>, "DAC"=→"DAC":refnum<visa-resource-name>, "DAC number"=→"DAC number":u8, "ITC signal"=→"ITC ref":T1)  [unwired: 2 out]
  "Nb Sweep Indicator" <- 1 ("Nb Sweep Indicator")
  "Nb Loop Indicator" <- 0.0 ("Nb Sweep Indicator")
